vi "AddStatusNotifier.vi"(8 "error in (no error)":errorcluster, 10 "Status Notifier":refnum<notifier>, 11 "MicroscopeController in":refnum<class "MicroscopeController.lvclass">) -> (0 "error out":errorcluster, 3 "MicroscopeController out":refnum<class "MicroscopeController.lvclass">)   [LabVIEW 2020, in "MicroscopeController.lvlib" / "MicroscopeController.lvclass"]
uses:
  MicroscopeController.lvclass
  MicroscopeController.lvclass/MicroscopeController.ctl
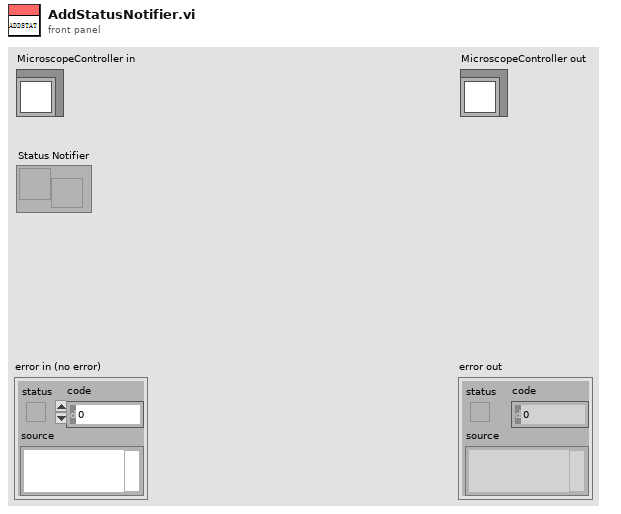
[diagram p1: front panel]
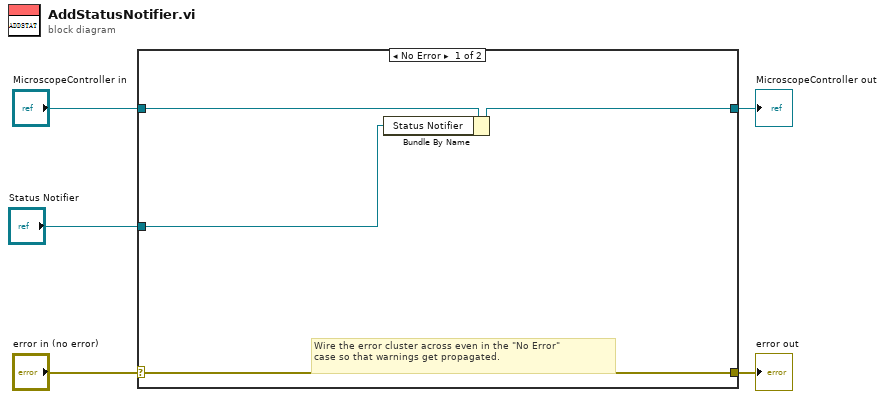
[diagram p0: block diagram]
diagram:
  n1 = case shown="No Error" "error in (no error)" {
    selector: "error in (no error)" -> [w8 w11]
    tunnel: [w8 w11] -> w4
    tunnel: [w7 w10] -> w2
    tunnel: "MicroscopeController in" -> [w9 w10]
    tunnel: "Status Notifier" -> [w6 _]
    frame No Error {
      # "Wire the error cluster across even in the \"No Error\"\ncase so that warnings get propagated."
      n2 = Bundle By Name(cluster=w9, "Status Notifier"=w6) -> (w7:refnum<class "MicroscopeController.lvclass">)
    }
    frame Error {
    }
  }
  "error out" <- w4
  "MicroscopeController out" <- w2
